vi "LeftDrivePID.vi"(11 "Time Delay Milli":u32) -> ()   [LabVIEW 2012]
uses:
  System Set Points and States.vi
  <vilib>/addons/control/pid/pid.llb/PID (DBL).vi
  <vilib>/Rock Robotics/WPI/RobotDrive/WPI_RobotDriveGetSetRefNum.vi
  <vilib>/addons/control/pid/NI_PID_pid.lvlib
panel:
  out "Stable":bool
  out "Speed Error":cluster{dbl, dbl, dbl[]}(graph)
  out "Output":dbl
  in  "Graph time interval  in seconds":dbl
  out "Drive Speed":cluster{dbl, dbl, dbl[]}(graph)
  out "RPM Error":dbl
  out "Encoder Speed":dbl
  in  "D":dbl=0.001
  in  "I":dbl=0.05
  in  "P":dbl=0.0025 step=0.001
  out "Encoder Set Speed":dbl
  # "These Work\n0.0025\n0.05\n0.001"
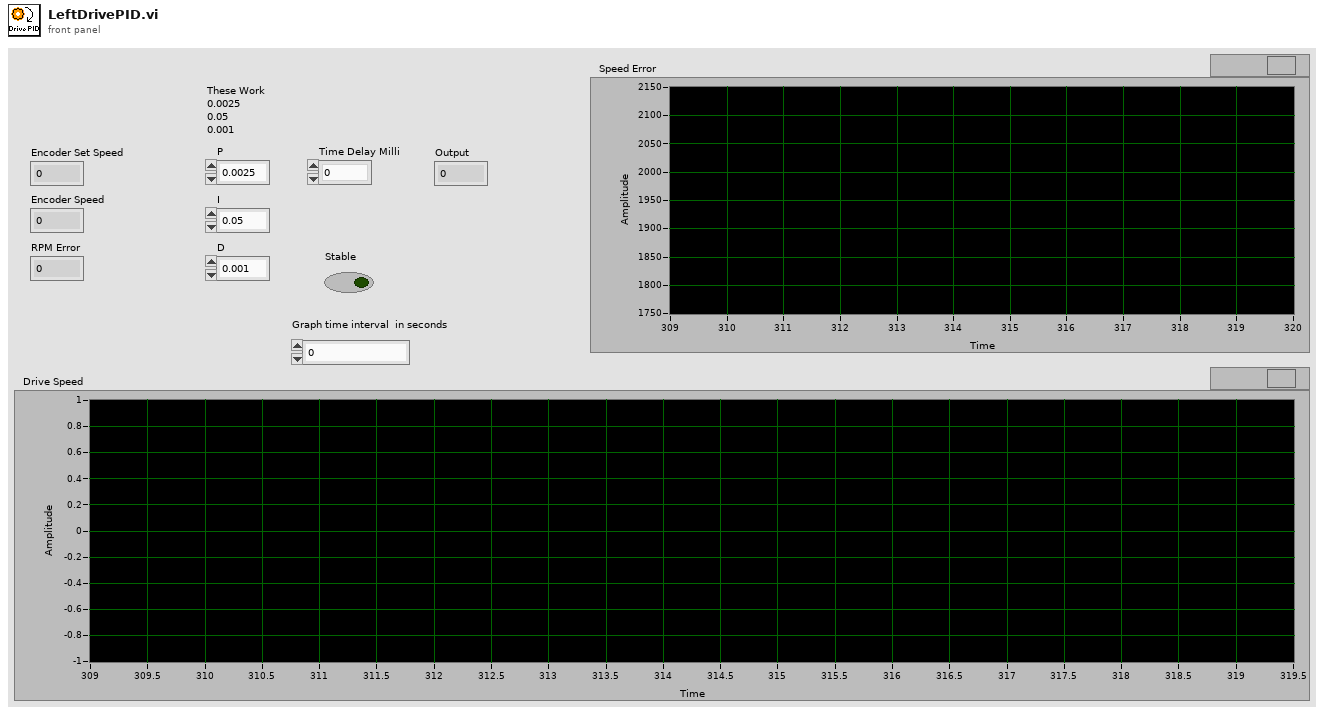
[diagram p1: front panel]
types:
  T1 = typedef "WPI_EncoderDevRef.ctl" = cluster{"DevStatus":errorcluster, "EncoderIndex":T2, "CounterIndex":T3, "DistancePerCount":dbl, "Decoding Type":T4}
  T2 = typedef "FPGA_EncoderIdx.ctl" = enum8{"Enc 0", "Enc 1", "Enc 2", "Enc 3", "Invalid"}
  T3 = typedef "FPGA_CounterCtrSystemIndex.ctl" = enum8{"Ctr 0", "Ctr 1", "Ctr 2", "Ctr 3", "Ctr 4", "Ctr 5", "Ctr 6", "Ctr 7", "Invalid"}
  T4 = typedef "WPI_EncoderType.ctl" = enum16{"1x", "2x", "4x"}
  T5 = typedef "WPI_RobotDriveDevRef.ctl" = cluster{"DevStatus":errorcluster, "Motors[]":T6[], "Square Inputs":bool, "Max Output":dbl, "Isochronous":bool}
  T6 = typedef "WPI_MotorControlDeviceRef.ctl" = cluster{"DeviceStatus":errorcluster, "Type":enum16{"PWM", "CAN"}, "PWM":cluster{"Digital Module":T7, "PWM Channel":T8, "DeadBand":T9}, "CAN":cluster{"Device Number":u8, "Control Mode":T10, "Semaphore":T11, "Max Vout":dbl}, "Invert":bool, "TransformRef":T12, "InvTransformRef":T12}
  T7 = typedef "FPGA_TypedefDigitalModule.ctl" = enum16{"Digital Module 1", "Digital Module 2"}
  T8 = typedef "FPGA_DIOPWMChannel.ctl" = enum8{"PWM 1", "PWM 2", "PWM 3", "PWM 4", "PWM 5", "PWM 6", "PWM 7", "PWM 8", "PWM 9", "PWM 10", "Invalid"}
  T9 = typedef "WPI_PWMDeadband.ctl" = cluster{"Name":string, "maxPositivePwm":i32, "minPositivePwm":i32, "centerPwm":i32, "maxNegativePwm":i32, "minNegativePwm":i32, "angularRange":u16}
  T10 = typedef "WPI_CANJaguar_ControlMode.ctl" = enum8{"Percent VBus", "Current", "Speed", "Position", "Voltage"}
  T11 = typedef "Semaphore RefNum" = refnum<k1>
  T12 = typedef "WPI_PWMTransform_ConPane.ctl" = refnum<vi>
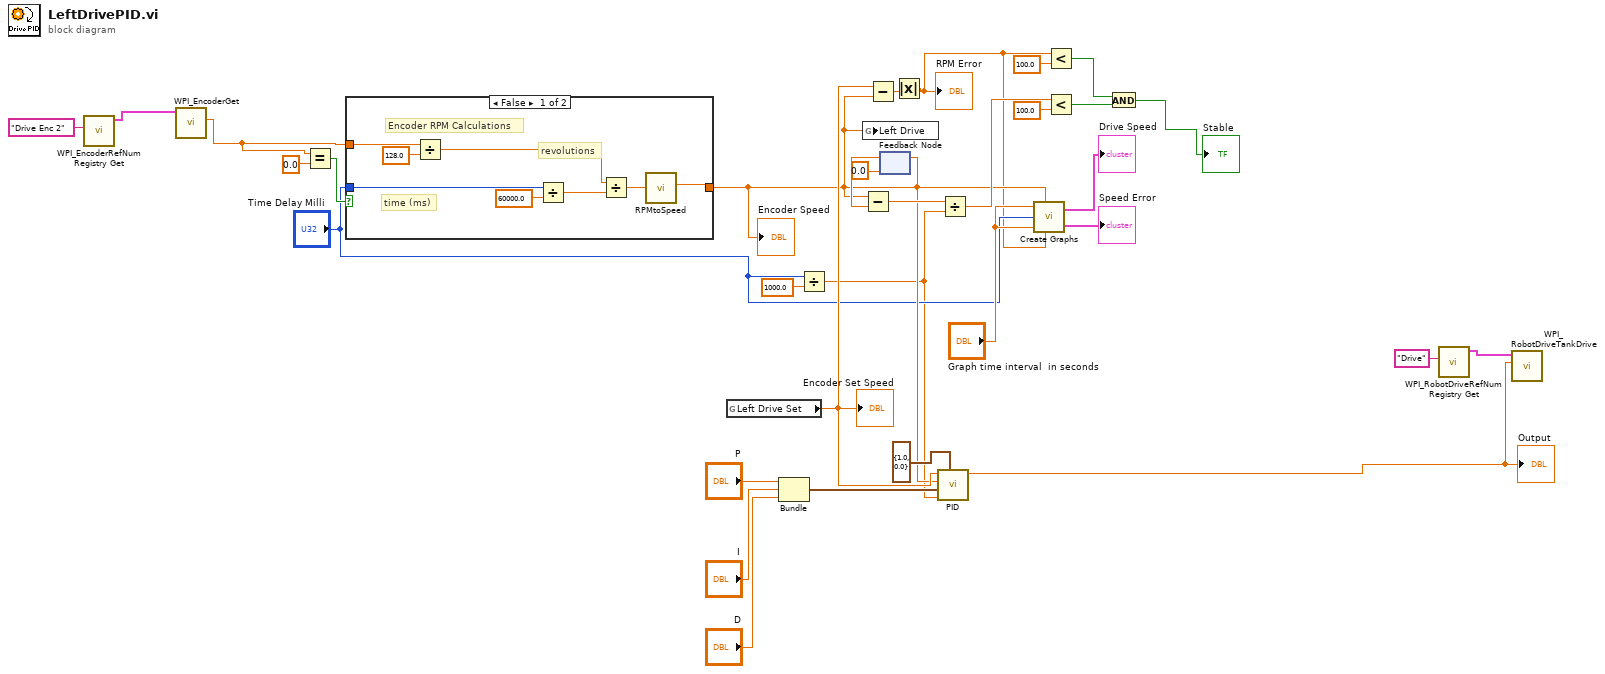
[diagram p0: block diagram]
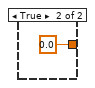
[diagram p2: hidden frame]
diagram:
  n1 = call <vilib>:"WPI_EncoderRefNum Registry Get.vi"("refnum name"="Drive Enc 2") -> ("EncoderDevRef"=w4:T1)  [unwired: 9 in, 1 out]
  n2 = call <vilib>:"WPI_EncoderGet.vi"("EncoderDevRef"=w4) -> ("Distance"=w5:dbl)  [unwired: 5 in, 5 out]
  n3 = Equal?(x=w5, y=0.0) -> (x = y?=w25:bool)
  n4 = case shown="False" w25 {
    tunnel: [w33 0.0] -> w13
    tunnel: w5 -> [w40 _]
    tunnel: "Time Delay Milli" -> [w38 _]
    frame False {
      # "time (ms)"
      # "revolutions"
      # "Encoder RPM Calculations"
      n5 = Divide(x=w40, y=128.0) -> (x/y=w39:dbl)
      n6 = Divide(x=w38, y=60000.0) -> (x/y=w36:dbl)
      n7 = Divide(x=w39, y=w36) -> (x/y=w34:dbl)
      n8 = call "RPMtoSpeed.vi"("RPM"=w34) -> ("Speed"=w33:dbl)  [unwired: 10 in]
    }
    frame True {
    }
  }
  "Encoder Speed" <- w13
  n9 = global read "System Set Points and States.vi" "Left Drive Set"() -> (w27:dbl)
  "Encoder Set Speed" <- w27
  n10 = Bundle("P"="P", "I"="I", "D"="D") -> (w28:cluster{"P":dbl, "I":dbl, "D":dbl})  [unwired: 1 in]
  n11 = Divide(x="Time Delay Milli", y=1000.0) -> (x/y=w9:dbl)
  n12 = global write "System Set Points and States.vi" "Left Drive"(w13) -> ()
  n13 = Subtract(x=w27, y=w13) -> (x-y=w7:dbl)
  n14 = feedback-in #1(w13) -> ()
  n15 = feedback #1(0.0) -> (w23:dbl)
  n16 = Subtract(x=w13, y=w23) -> (x-y=w22:dbl)
  n17 = Absolute Value(x=w7) -> (abs(x)=w6:dbl)
  "RPM Error" <- w6
  n18 = call-poly <vilib>:"PID.vi"("output range"=cluster{"output high":dbl, "output low":dbl} {"output high"=1.0, "output low"=0.0}, "dt (s)"=w9, "PID gains"=w28, "process variable"=w13, "setpoint"=w27) -> ("output"=w24:dbl)  [unwired: 5 in, 1 out]
  "Output" <- w24
  n19 = Divide(x=w22, y=w9) -> (x/y=w21:dbl)
  n20 = call "Create Graphs.vi"("Speed Graph Time"="Graph time interval  in seconds", "Speed"=w13, "Time Delay"="Time Delay Milli", "Error Graph Time"="Graph time interval  in seconds", "Error"=w6) -> ("Speed"=→"Drive Speed":cluster{dbl, dbl, dbl[]}, "Error"=→"Speed Error":cluster{dbl, dbl, dbl[]})
  n21 = Less?(x=w6, y=100.0) -> (x < y?=w17:bool)
  n22 = Less?(x=w21, y=100.0) -> (x < y?=w19:bool)
  n23 = And(x=w17, y=w19) -> (x .and. y?=→"Stable":bool)
  n24 = call <vilib>:"WPI_RobotDriveRefNum Registry Get.vi"("refnum name"="Drive") -> ("RobotDriveDevRef"=w2:T5)  [unwired: 9 in, 1 out]
  n25 = call <vilib>:"WPI_RobotDriveTankDrive.vi"("Left axis value"=w24, "RobotDriveDevRef"=w2) -> ()  [unwired: 7 in, 3 out]
